vi "Get Valve From Name.vi"(10 "Name":string) -> (0 "Valid?":bool, 2 "Valve":T1)   [LabVIEW 2015]
uses:
  Valve Name Enum.ctl
panel:
  in  "Enum":T1
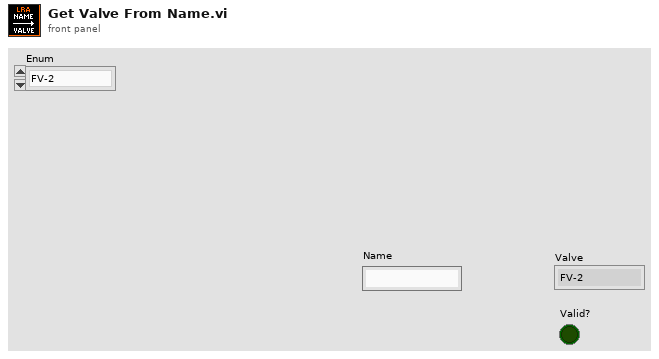
[diagram p1: front panel]
types:
  T1 = typedef "Valve Name Enum.ctl" = enum16{"FV-2", "FV-3", "FV-4", "OV-2", "OV-3", "OV-4", "NV-2", "COMP"}
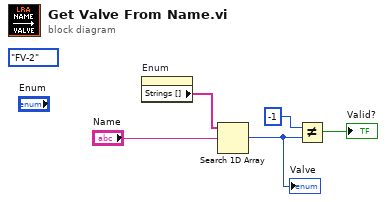
[diagram p0: block diagram]
diagram:
  (unwired) Valve_Name_Enum."FV-2" ("Enum")
  n1 = property on="Enum" class="Enum (strict)"() -> ("Strings []"=w5:string[])  [unwired: 2 in, 2 out]
  n2 = Search 1D Array(1D array=w5, element="Name") -> (index of element=w1:i32)  [unwired: 1 in]
  "Valve" <- w1
  n3 = Not Equal?(x=-1, y=w1) -> (x != y?=→"Valid?":bool)
